vi "Parse.vi"(8 "error in (no error)":errorcluster, 10 "Data String":string, 11 "Multi Parser in":refnum<class "Multi Sentence Parser.lvclass">) -> (0 "error out":errorcluster, 2 "Data Values":dbl[](array[numeric]), 3 "Multi Parser out":refnum<class "Multi Sentence Parser.lvclass">)   [LabVIEW 2018, in "Multi Sentence Parser.lvclass"]
doc: "Multi Sentence Parser.lvclass:Parse.vi\n\nThis VI parses multiple strings read from an instrument as input and returns an array of channel values.\n\nInstrument Communication Module Version 1.0\nOctober, 2018 Original Code Consulting David Thomson\n www.originalcode.com"
uses:
  Multi Sentence Parser.lvclass
  Multi Sentence Parser.lvclass/Multi Sentence Parser.ctl
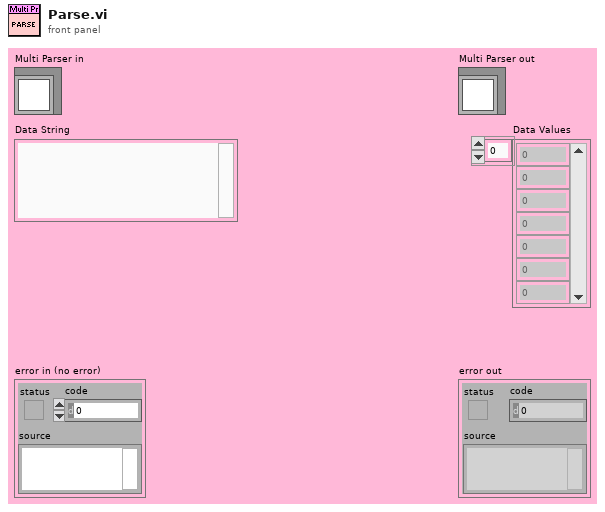
[diagram p1: front panel]
types:
  T1 = cluster{"Sentence ID":string, "Format String":string, "Channels":string[], "Enabled":bool[], "Ignore Missing Sentences?":bool}[]
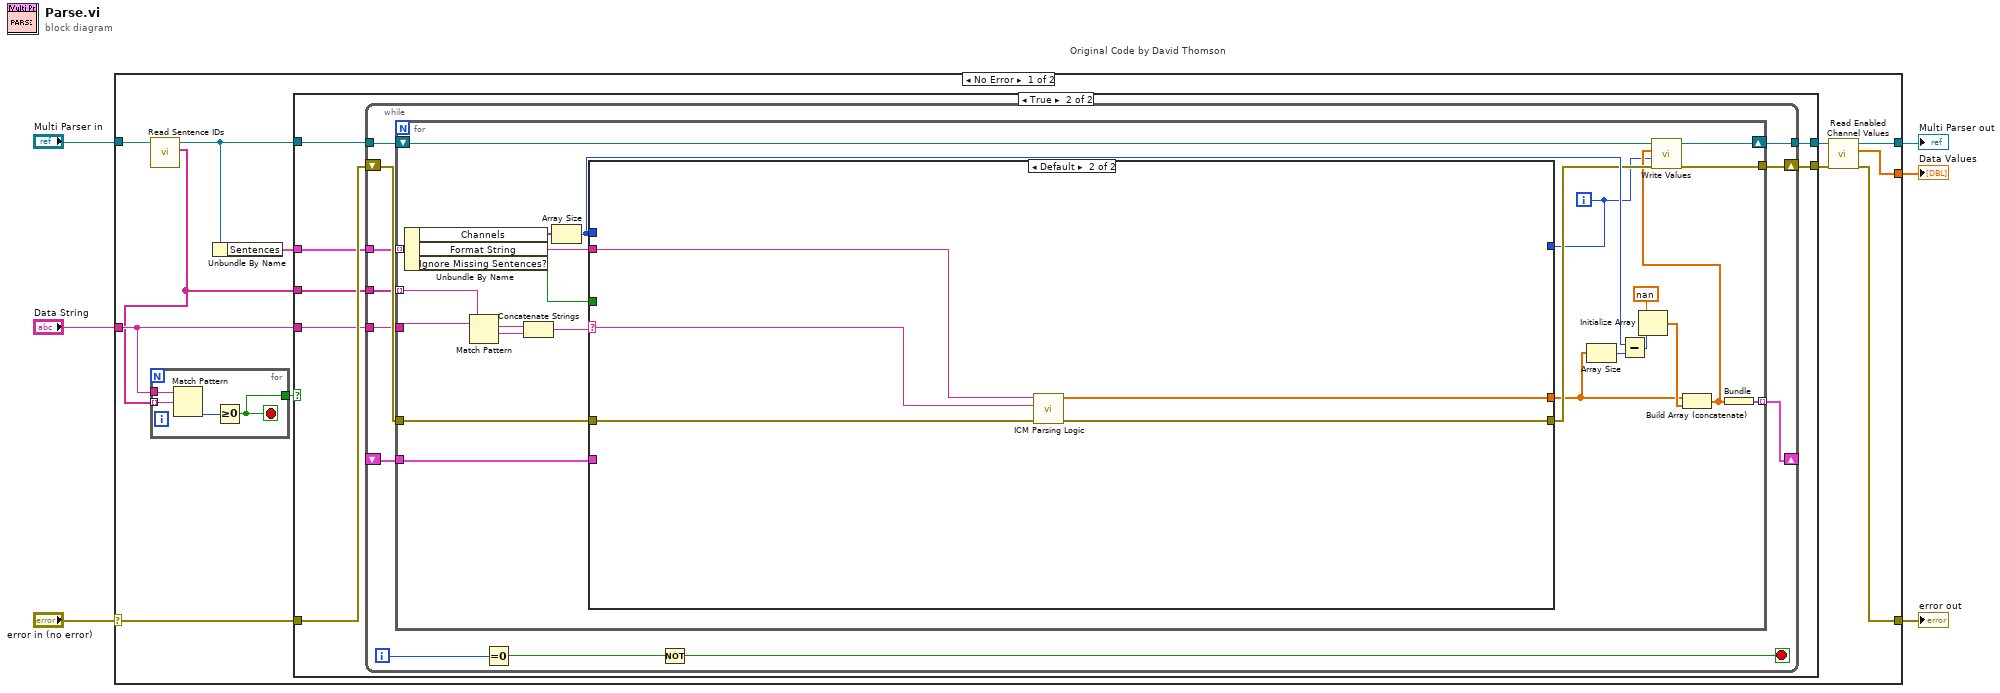
[diagram p0: block diagram]
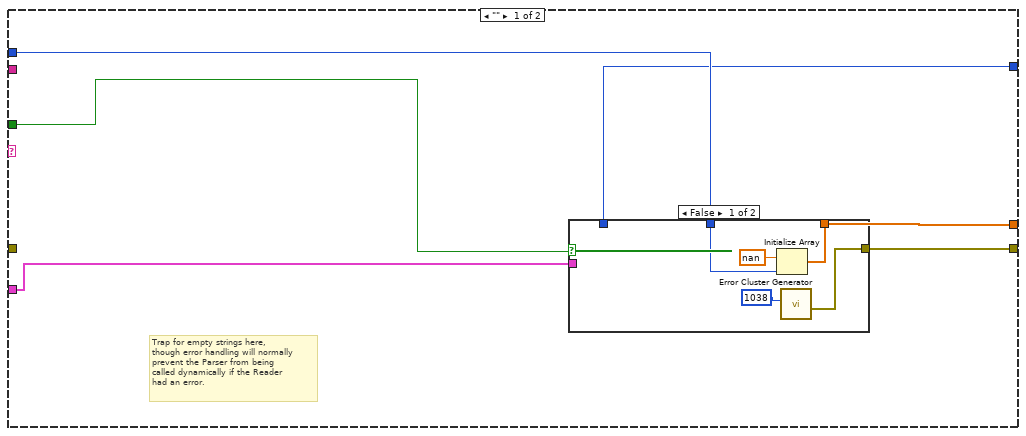
[diagram p3: hidden frame]
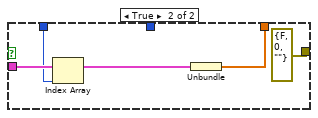
[diagram p4: hidden frame]
diagram:
  n1 = case "Original Code by David Thomson" shown="No Error" "error in (no error)" {
    selector: "error in (no error)" -> [w18 w90]
    tunnel: [w14 w90] -> w5
    tunnel: "Multi Parser in" -> [w17 w89]
    tunnel: "Data String" -> [w16 _]
    tunnel: [w11 _] -> w2
    tunnel: [w10 w89] -> w1
    frame No Error {
      n2 = call-dynamic "Read Sentence IDs.vi"("Multi Parser in"=w17) -> ("Sentence IDs"=w8:string[], "Multi Parser out"=w15:refnum<class "Multi Sentence Parser.lvclass">)  [unwired: 8 in, 1 out]
      n3 = for {
        tunnel: w8 -> [w87] mode=indexing
        tunnel: w16 -> [w88]
        tunnel: [w85] -> w7
        stop <- w85 stop-if-true
        n4 = Match Pattern(string=w88, regular expression=w87) -> (offset past match=w86:i32)  [unwired: 1 in, 3 out]
        n5 = Greater Or Equal To 0?(x=w86) -> (x >= 0?=w85:bool)
      }
      n6 = Unbundle By Name(w15) -> ("Sentences"=w13:T1)
      n7 = case shown="True" w7 {
        tunnel: w18 -> [w20 w27]
        tunnel: [w20 w24] -> w12
        tunnel: w16 -> [_ w26]
        tunnel: w13 -> [_ w21]
        tunnel: w15 -> [w19 w25]
        tunnel: [w19 w23] -> w9
        tunnel: w8 -> [_ w22]
        frame False {
        }
        frame True {
          n8 = while {
            tunnel: w26 -> [w38]
            tunnel: w21 -> [w37]
            tunnel: w22 -> [w33]
            shift-right: [w35] -> w24
            shift-left: w27 -> [w39]
            shift-right: [w32] -> _
            shift-left: _ -> [w31]
            tunnel: w25 -> [w36]
            tunnel: [w34] -> w23
            i -> [w30]
            stop <- w28 stop-if-true
            n9 = for {
              tunnel: w37 -> [w60] mode=indexing
              tunnel: w39 -> [w63]
              tunnel: [w52] -> w35
              tunnel: w38 -> [w50]
              tunnel: w33 -> [w49] mode=indexing
              tunnel: [w43] -> w32 mode=indexing
              tunnel: w31 -> [w42]
              shift-right: [w51] -> w34
              shift-left: w36 -> [w55]
              i -> [w41]
              n10 = Unbundle By Name(w60) -> ("Channels"=w62:string[], "Format String"=w40:string, "Ignore Missing Sentences?"=w45:bool)
              n11 = Match Pattern(string=w50, regular expression=w49) -> (match substring=w48:string, after substring=w47:string)  [unwired: 1 in, 2 out]
              n12 = Concatenate Strings(w48, w47) -> (w46:string)
              n13 = Array Size(array=w62) -> (size(s)=w61:i32)
              n14 = case shown="Default" w46 {
                selector: w46 -> [_ w81]
                tunnel: w63 -> [_ w84]
                tunnel: [w69 w83] -> w56
                tunnel: [w66 w82] -> w54
                tunnel: w61 -> [w65 _]
                tunnel: w45 -> [w68 _]
                tunnel: w42 -> [w67 _]
                tunnel: w41 -> [w64 _]
                tunnel: w40 -> [_ w80]
                frame "" {
                  # "Trap for empty strings here,\nthough error handling will normally\nprevent the Parser from being\ncalled dynamically if the Reader\nhad an error."
                  n15 = case shown="False" w68 {
                    tunnel: [w74 errorcluster {"status"=FALSE, "code"=0, "source"=""} ("error out")] -> w69
                    tunnel: w67 -> [_ w78]
                    tunnel: [w71 w77] -> w66
                    tunnel: w65 -> [w70 _]
                    tunnel: w64 -> [_ w75]
                    frame False {
                      n16 = Initialize Array(nan ("y"), w70) -> (w71:dbl[])
                      n17 = call "Error Cluster Generator.vi"("code"=1038) -> ("error out"=w74:errorcluster)  [unwired: 5 in, 1 out]
                    }
                    frame True {
                      n18 = Index Array(array=w78, index=w75) -> (element=w76:cluster{dbl[]})
                      n19 = Unbundle(w76) -> (w77:dbl[])
                    }
                  }
                }
                frame Default {
                  n20 = call "ICM Parsing Logic.vi"("error in (no error)"=w84, "Data String"=w81, "Format String"=w80) -> ("error out"=w83:errorcluster, "Data Values"=w82:dbl[])  [unwired: 7 in]
                }
              }
              n21 = Array Size(array=w54) -> (size(s)=w57:i32)
              n22 = Subtract(x=w61, y=w57) -> (x-y=w58:i32)
              n23 = Initialize Array(nan ("y"), w58) -> (w59:dbl[])
              n24 = Build Array (concatenate)(w54, w59) -> (w44:dbl[])
              n25 = call-dynamic "Write Values.vi"("error in (no error)"=w56, "Sentence Index"=w41, "Values"=w44, "Multi Parser in"=w55) -> ("error out"=w52:errorcluster, "Multi Parser out"=w51:refnum<class "Multi Sentence Parser.lvclass">)  [unwired: 6 in]
              n26 = Bundle(w44) -> (w43:cluster{dbl[]})  [unwired: 1 in]
            }
            n27 = Equal To 0?(x=w30) -> (x = 0?=w29:bool)
            n28 = Not(x=w29) -> (.not. x?=w28:bool)
          }
        }
      }
      n29 = call-dynamic "Read Enabled Channel Values.vi"("error in (no error)"=w12, "Multi Parser in"=w9) -> ("error out"=w14:errorcluster, "Enabled Values"=w11:dbl[], "Multi Parser out"=w10:refnum<class "Multi Sentence Parser.lvclass">)  [unwired: 7 in]
    }
    frame Error {
    }
  }
  "error out" <- w5
  "Multi Parser out" <- w1
  "Data Values" <- w2
